vi "get peak location.vi"(9 "Peak index":i32, 10 "Threshold":dbl, 11 "In":dbl[](array[numeric])) -> (3 "Numeric":dbl)   [LabVIEW 2014]
uses:
  <vilib>/Analysis/NI_AAL_SigProc.lvlib
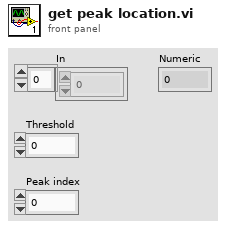
[diagram p1: front panel]
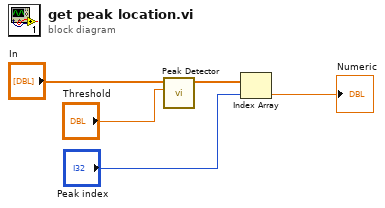
[diagram p0: block diagram]
diagram:
  n1 = call <vilib>:"Peak Detector.vi"("threshold"="Threshold", "X"="In") -> ("Locations"=w2:dbl[])  [unwired: 5 in, 4 out]
  n2 = Index Array(array=w2, index="Peak index") -> (element=→"Numeric":dbl)
